vi "CANOpen_Main_Set All Node States.vi"(8 "error in (no error)":errorcluster, 9 "command":u16(ring)=128 items=["start remote node"=1, "stop remote node"=2, "enter pre-operational"=128, "reset node"=129, "reset communication"=130], 10 "Nodes":T1[](array[typedef]) {"NMT"."Node init static SDO state" items=["start remote node"=1, "enter pre-operational"=128]; "NMT"."Node run state" items=["start remote node"=1, "stop remote node"=2, "enter pre-operational"=128, "reset node"=129, "reset communication"=130]; "Dynamic SDOs"."Sub-Index (0)" format="%.0x"; "Dynamic SDOs"."Object Index" format="%.0x"; "Dynamic SDOs"."Block Data" format="%.0x"; "RPDOs"."PDO Channel" items=["PDO 1", "PDO 2", "PDO 3", "PDO 4"]; "RPDOs"."Parameters"."Bit Offset" max=8 step=1; "RPDOs"."Parameters"."Byte Offset" max=8 step=1; "TPDOs"."PDO Channel" items=["PDO 1", "PDO 2", "PDO 3", "PDO 4"]; "TPDOs"."Parameters"."Bit Offset" max=8 step=1; "TPDOs"."Parameters"."Byte Offset" max=8 step=1; "SDOs"."Sub-Index (0)" format="%.0x"; "SDOs"."Object Index" format="%.0x"; "SDOs"."Block Data" format="%.0x"}, 11 "interface object":refnum<k20>) -> (0 "error out":errorcluster, 3 "interface object out":refnum<k20>)   [LabVIEW 2021, in "CANOpen Addon Engine.lvlib"]
uses:
  CANOpen Addon Engine.lvlib
  SubVIS/CANOpen_Node Message Settings.ctl
  Shared/CANOpen_PDO Settings.ctl
  Shared/CANOpen_PDO Parameter Settings.ctl
  Shared/CANOpen_PDO Data Type.ctl
  System Explorer/SubVIs/CANopen Byte Order.ctl
  Shared/CANOpen_SDO Settings.ctl
  SubVIS/CANOpen_NMT Settings.ctl
  CanOpen_NMT_Config.ctl
  CanOpen_NMT_Static detect.ctl
  Shared/CANOpen Addon Shared.lvlib
  System Explorer/CANOpen Addon System Explorer.lvlib
panel:
  # "LSB"
  # "MSB"
  # "LSB"
  # "MSB"
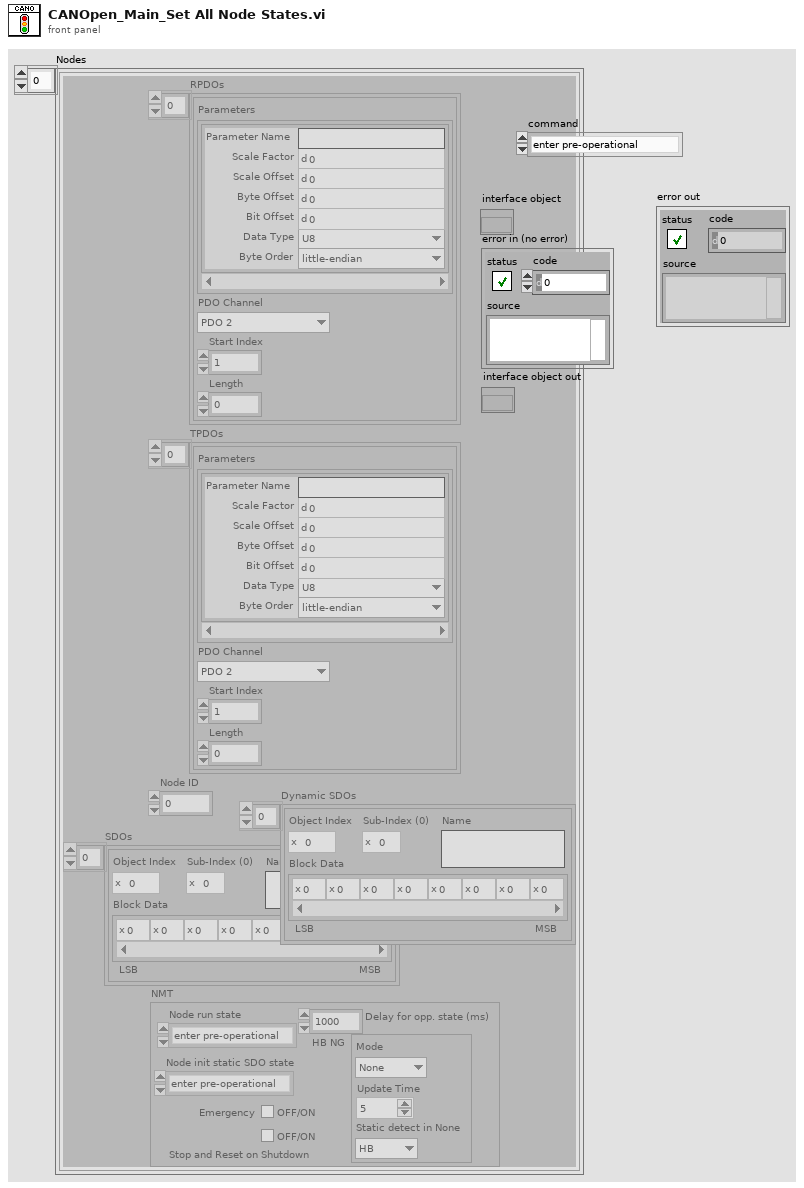
[diagram p1: front panel]
types:
  T1 = typedef "CANOpen Addon Engine.lvlib/CANOpen_Node Message Settings.ctl" = cluster{"RPDOs":T2[], "TPDOs":T2[], "Node ID":u8, "SDOs":T6[], "Dynamic SDOs":T6[], "NMT":T7}
  T2 = typedef "CANOpen Addon Shared.lvlib/CANOpen_PDO Settings.ctl" = cluster{"Parameters":T3[], "PDO Channel":u8, "Start Index":u32, "Length":u32}
  T3 = typedef "CANOpen Addon Shared.lvlib/CANOpen_PDO Parameter Settings.ctl" = cluster{"Parameter Name":string, "Scale Factor":dbl, "Scale Offset":dbl, "Byte Offset":u8, "Bit Offset":u8, "Data Type":T4, "Byte Order":T5}
  T4 = typedef "CANOpen Addon Shared.lvlib/CANOpen_PDO Data Type.ctl" = enum16{"U8", "U16", "U32", "I8", "I16", "I32", "Single", "Double", "Boolean"}
  T5 = typedef "CANOpen Addon System Explorer.lvlib/CANopen Byte Order.ctl" = enum16{"big-endian network order", "little-endian"}
  T6 = typedef "CANOpen Addon Shared.lvlib/CANOpen_SDO Settings.ctl" = cluster{"Object Index":u16, "Sub-Index (0)":u8, "Block Data":u8[], "Name":string}
  T7 = typedef "CANOpen Addon Engine.lvlib/CANOpen_NMT Settings.ctl" = cluster{"Node run state":u16, "Emergency":bool, "HB NG":T8, "Delay for opp. state (ms)":dbl, "Node init static SDO state":u16, "Stop and Reset on Shutdown":bool}
  T8 = typedef "CANOpen Addon Engine.lvlib/CanOpen_NMT_Config.ctl" = cluster{"Mode":T9, "Update Time":u16, "Static detect in None":T9}
  T9 = typedef "CANOpen Addon Engine.lvlib/CanOpen_NMT_Static detect.ctl" = enum16{"None", "HB", "NG"}
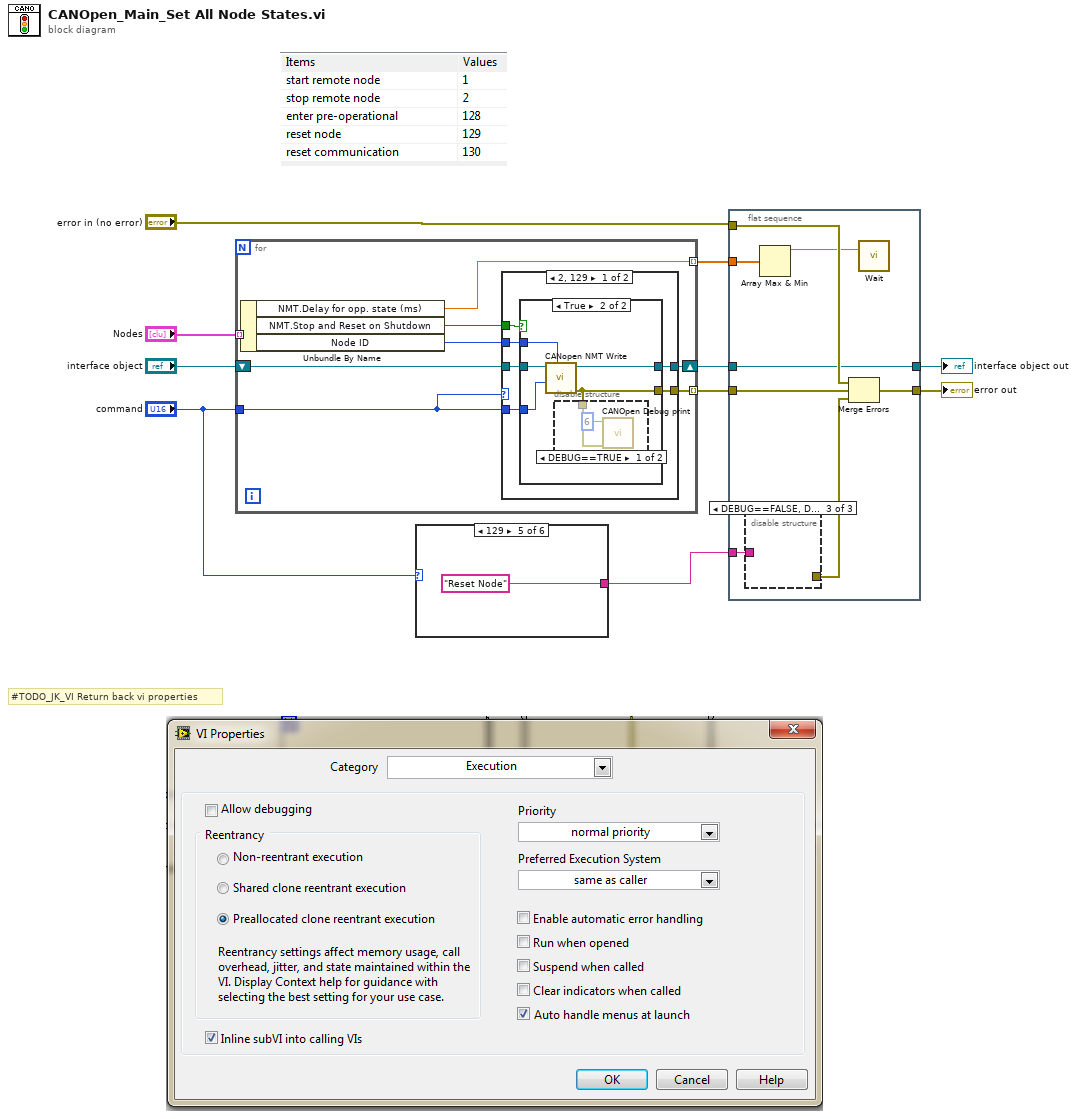
[diagram p0: block diagram]
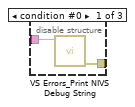
[diagram p2: hidden frame]
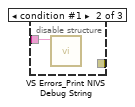
[diagram p3: hidden frame]
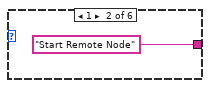
[diagram p5: hidden frame]
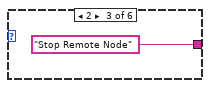
[diagram p6: hidden frame]
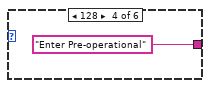
[diagram p7: hidden frame]
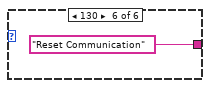
[diagram p8: hidden frame]
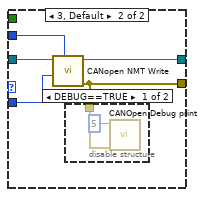
[diagram p11: hidden frame]
diagram:
  # "#TODO_JK_VI Return back vi properties"
  n1 = for {
    shift-right: [w17] -> w3
    shift-left: "interface object" -> [w18]
    tunnel: "Nodes" -> [w16] mode=indexing
    tunnel: "command" -> [w13]
    tunnel: [w14] -> w6 mode=indexing
    tunnel: [w11] -> w2 mode=indexing
    n2 = Unbundle By Name(w16) -> ("NMT.Delay for opp. state (ms)"=w11:dbl, "NMT.Stop and Reset on Shutdown"=w12:bool, "Node ID"=w15:u8)
    n3 = case shown="2, 129" w13 {
      tunnel: w18 -> [w24 w37]
      tunnel: [w23 w36] -> w17
      tunnel: w15 -> [w22 w35]
      tunnel: w13 -> [w21 w34]
      tunnel: [w20 w33] -> w14
      tunnel: w12 -> [w19 _]
      frame 2, 129 {
        n4 = case shown="True" w19 {
          tunnel: w24 -> [w25 w30]
          tunnel: [w25 w29] -> w23
          tunnel: w22 -> [_ w28]
          tunnel: w21 -> [_ w27]
          tunnel: [_ w26] -> w20
          frame False {
          }
          frame True {
            n5 = call <vilib>:"CANopen NMT Write.vi"("node-ID (0)"=w28, "command"=w27, "interface object in"=w30) -> ("error out"=w26:errorcluster, "interface object out"=w29:refnum<k20>)  [unwired: 7 in]
            n6 = disable-structure shown="DEBUG==TRUE" {
              disable-tunnel: w26 -> [w32 _]
              frame condition #0 {
                n7 = call "CANOpen Debug print.vi"("error in (no error)"=w32, "ID"=u8 6) -> ()  [unwired: 10 in]
              }
              frame condition #1 (active) {
              }
            }
          }
        }
      }
      frame 3, Default {
        n8 = call <vilib>:"CANopen NMT Write.vi"("node-ID (0)"=w35, "command"=w34, "interface object in"=w37) -> ("error out"=w33:errorcluster, "interface object out"=w36:refnum<k20>)  [unwired: 7 in]
        n9 = disable-structure shown="DEBUG==TRUE" {
          disable-tunnel: w33 -> [w38 _]
          frame condition #0 {
            n10 = call "CANOpen Debug print.vi"("error in (no error)"=w38, "ID"=u8 5) -> ()  [unwired: 10 in]
          }
          frame condition #1 (active) {
          }
        }
      }
    }
  }
  n11 = case shown="129" "command" {
    tunnel: [_ "Start Remote Node" "Stop Remote Node" "Enter Pre-operational" "Reset Node" "Reset Communication"] -> w1
    frame Default {
    }
    frame 1 {
    }
    frame 2 {
    }
    frame 128 {
    }
    frame 129 {
    }
    frame 130 {
    }
  }
  n12 = flat-sequence {
    tunnel: [w49] -> w8
    tunnel: w1 -> [w52]
    tunnel: w6 -> [w51]
    tunnel: "error in (no error)" -> [w48]
    tunnel: [w47] -> w4
    tunnel: w3 -> [w47]
    tunnel: w2 -> [w46]
    frame #0 {
      n13 = disable-structure shown="DEBUG==FALSE, Default" {
        disable-tunnel: w52 -> [w54 w55 _]
        disable-tunnel: [w53 _ _] -> w50
        frame condition #0 {
          n14 = call "VS Errors_Print NIVS Debug String.vi"("Debug String"=w54) -> ("error out"=w53:errorcluster)  [unwired: 9 in]
        }
        frame condition #1 {
          n15 = call "VS Errors_Print NIVS Debug String.vi"("Debug String"=w55) -> ()  [unwired: 9 in, 1 out]
        }
        frame condition #2 (active) {
        }
      }
      n16 = Array Max & Min(array=w46) -> (max value=w45:dbl)  [unwired: 3 out]
      n17 = Merge Errors(w48, w51, w50) -> (w49:errorcluster)
      n18 = call "Wait"("Count(mSec)"=w45) -> ()  [unwired: 1 out]
    }
  }
  "error out" <- w8
  "interface object out" <- w4
